vi "Vertical Fill Slide.vi"() -> ()   [LabVIEW 2023]
doc: "This VI demonstrates how property nodes can be used to change the fill color in a Vertical Fill Slide indicator. It decides the color of the fill based on the value of the Vertical Fill Slide control."
panel:
  in  "Stop":bool
  out "Vertical Fill Slide Indicator":dbl(slide) scale=0.0..100.0
  in  "Vertical Fill Slide Control":dbl(slide) scale=0.0..100.0
  # "Overview: Demonstrates the use of the Vertical Fill Slide numeric control.\nInstructions:\n1. Run the VI.\n2. Change the value of the Vertical Fill Slide Control, either by clicking and dragging within the fill area, or changing the value of the Digital Display. Notice that the fill color of the Vertical Fill Slide Indicator will change depending on its value.\n3. Click Stop to stop the VI."
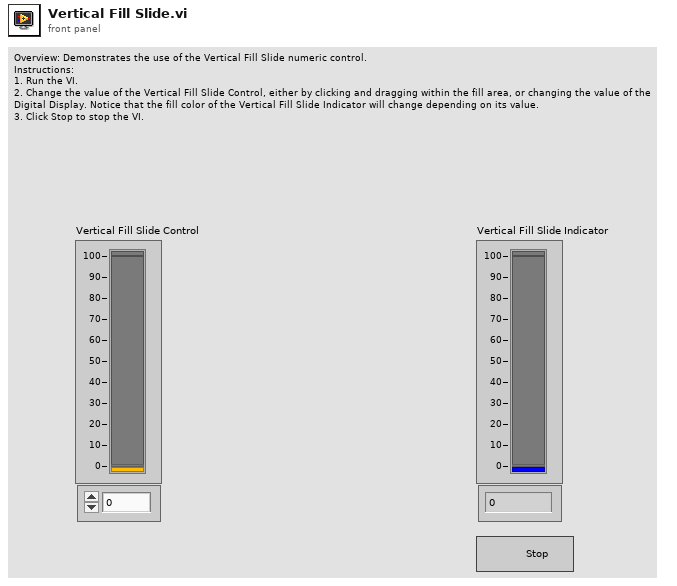
[diagram p1: front panel]
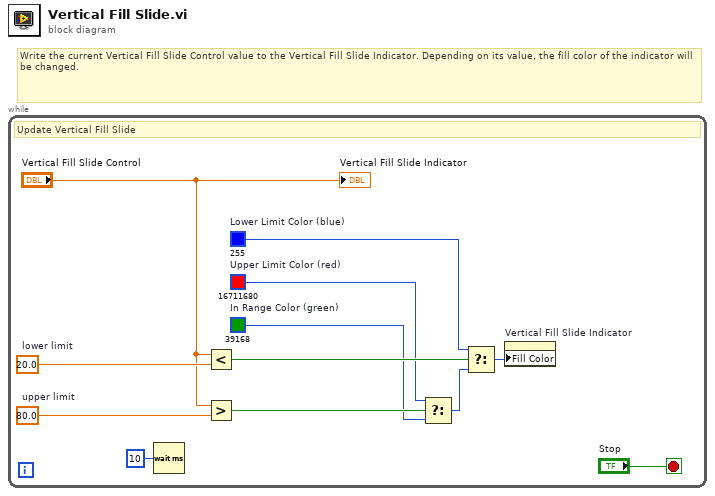
[diagram p0: block diagram]
diagram:
  # "Write the current Vertical Fill Slide Control value to the Vertical Fill Slide Indicator. Depending on its value, the fill color of the indicator will be changed."
  n1 = while {
    stop <- "Stop" stop-if-true
    w2 = u32 39168  # In Range Color (green)
    w5 = u32 255  # Lower Limit Color (blue)
    w1 = u32 16711680  # Upper Limit Color (red)
    w8 = 80.0  # upper limit
    w11 = 20.0  # lower limit
    # "Update Vertical Fill Slide"
    n2 = Wait (ms)(milliseconds to wait=u32 10) -> ()  [unwired: 1 out]
    n3 = Less?(x="Vertical Fill Slide Control", y=w11) -> (x < y?=w10:bool)
    n4 = Greater?(x="Vertical Fill Slide Control", y=w8) -> (0:w7:bool)
    n5 = Select(t=w1, s=w7, f=w2) -> (s? t:f=w4:u32)
    n6 = Select(t=w5, s=w10, f=w4) -> (s? t:f=w3:u32)
    n7 = property on="Vertical Fill Slide Indicator" class="Slide (strict)"("Fill Color"=w3) -> ()  [unwired: 2 in, 2 out]
    "Vertical Fill Slide Indicator" <- "Vertical Fill Slide Control"
  }
